vi "Test U8 Comm.vi"() -> ()   [LabVIEW 2021]
uses:
  ChannelCommon/typedef/FIFO Config.ctl
  ChannelCommon/ChannelCommon.lvlib
  CIFChannels/Typedef/Direction.ctl
  CIFChannels/CIFChannels.lvclass
  CIF_CIPC_Fifo_DAQ.lvclass
  ChannelCommon/typedef/TimeStamps.ctl
panel:
  out "status":string
  out "pass":bool
  out "error out":errorcluster
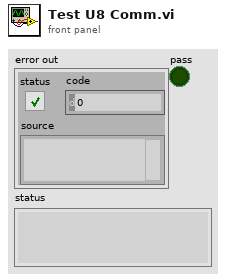
[diagram p1: front panel]
types:
  T1 = typedef "CIFChannels.lvclass/Direction.ctl" = enum16{"Publisher", "Subscriber"}
  T2 = typedef "ChannelCommon.lvlib/TimeStamps.ctl" = cluster{"ClockID":u8, "T0":i64, "T_Out":i64}
  T3 = typedef "ChannelCommon.lvlib/FIFO Config.ctl" = cluster{"Max Bytes/Msg":u64, "Max Msg/FIFO":u64, "Flags":u64}
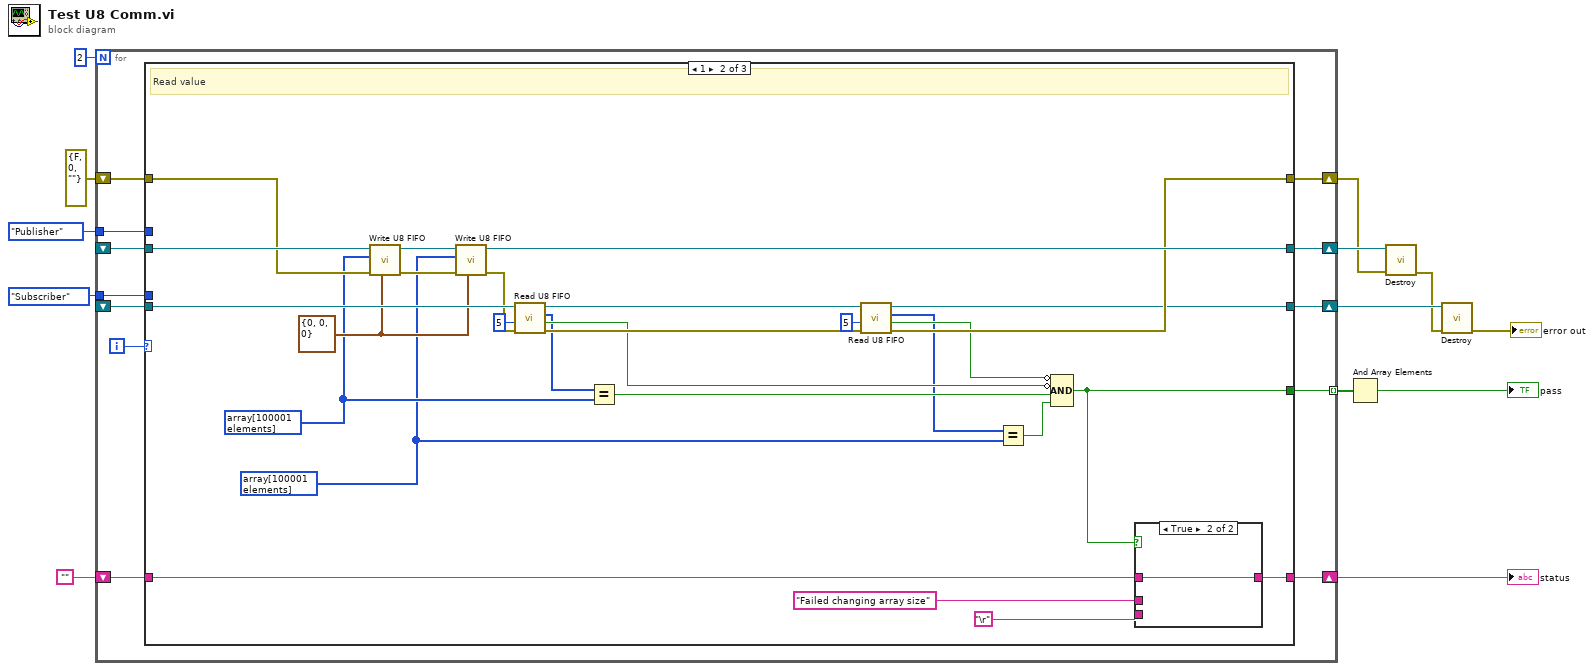
[diagram p0: block diagram]
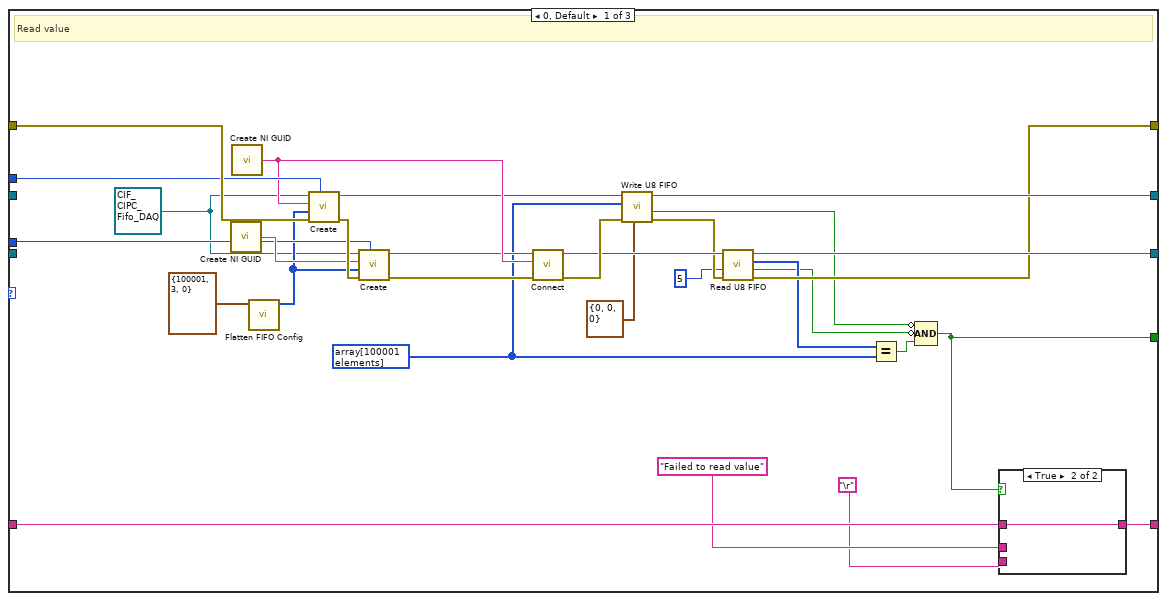
[diagram p2: hidden frame]
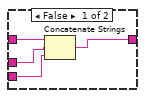
[diagram p3: hidden frame]
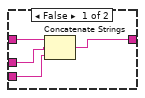
[diagram p4: hidden frame]
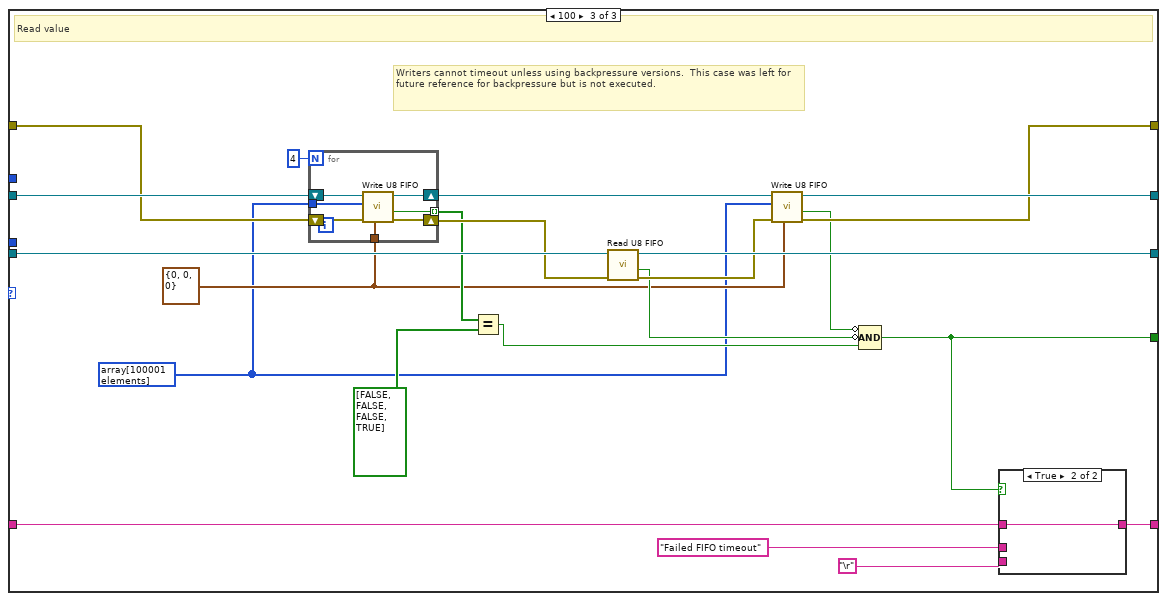
[diagram p5: hidden frame]
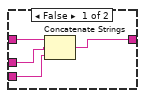
[diagram p6: hidden frame]
diagram:
  n1 = for {
    N: 2 -> [_]
    tunnel: [w25] -> w13 mode=indexing
    shift-right: [w23] -> w3
    shift-left: errorcluster {"status"=FALSE, "code"=0, "source"=""} ("error out") -> [w24]
    shift-right: [w20] -> w9
    shift-left: "" -> [w21]
    tunnel: Direction."Subscriber" ("Direction") -> [w19]
    tunnel: Direction."Publisher" ("Direction") -> [w18]
    shift-right: [w17] -> w5
    shift-left: _ -> [w15]
    shift-right: [w16] -> w4
    shift-left: _ -> [w14]
    i -> [w22]
    n2 = case shown="1" w22 {
      tunnel: [w50 w83 w95] -> w25
      tunnel: w24 -> [w48 w79 w109]
      tunnel: [w36 w72 w101] -> w23
      tunnel: w21 -> [w55 w87 w114]
      tunnel: [w54 w86 w113] -> w20
      tunnel: w19 -> [w46 _ _]
      tunnel: w18 -> [w45 _ _]
      tunnel: [w37 w69 w106] -> w17
      tunnel: [w39 w76 w104] -> w16
      tunnel: w14 -> [_ w80 w110]
      tunnel: w15 -> [_ w75 w107]
      frame 0, Default {
        w28 = refnum<class "CIF_CIPC_Fifo_DAQ.lvclass"> refnum ("CIF_CIPC_Fifo_U8.lvclass")
        w29 = u8[] array[100001 elements] ("U8 Data")
        # "Read value"
        n3 = call <vilib>:"Create NI GUID.vi"() -> ("NI GUID"=w47:string)
        n4 = call <vilib>:"Create NI GUID.vi"() -> ("NI GUID"=w43:string)
        n5 = call "Flatten FIFO Config.vi"("FIFO Config in"=T3 {"Max Bytes/Msg"=100001, "Max Msg/FIFO"=3, "Flags"=0}) -> ("Flattened FIFO Config"=w30:u8[])  [unwired: 10 in]
        n6 = call-dynamic "Create.vi"("Direction"=w45, "error in (no error)"=w48, "Custom Config Data"=w30, "Name"=w43, "CIFFIFO in"=w28) -> ("error out"=w49:errorcluster, "CIFFIFO out"=w26:refnum<class "CIF_CIPC_Fifo_DAQ.lvclass">)  [unwired: 5 in]
        n7 = call-dynamic "Create.vi"("Direction"=w46, "error in (no error)"=w49, "Custom Config Data"=w30, "Name"=w47, "CIFFIFO in"=w28) -> ("error out"=w42:errorcluster, "CIFFIFO out"=w41:refnum<class "CIF_CIPC_Fifo_DAQ.lvclass">)  [unwired: 5 in]
        n8 = call-dynamic "Connect.vi"("error in (no error)"=w42, "Connection Name"=w43, "CIFTag in"=w41) -> ("error out"=w40:errorcluster, "CIFTag out"=w38:refnum<class "CIF_CIPC_Fifo_DAQ.lvclass">)  [unwired: 7 in]
        n9 = call-dynamic "Write U8 FIFO.vi"("FIFO Timestamps"=T2 {"ClockID"=0, "T0"=0, "T_Out"=0}, "error in (no error)"=w40, "Data in"=w29, "CIFFIFO in"=w26) -> ("error out"=w35:errorcluster, "timed out?"=w34:bool, "CIFFIFO out"=w39:refnum<class "CIF_CIPC_Fifo_DAQ.lvclass">)  [unwired: 4 in, 1 out]
        n10 = call-dynamic "Read U8 FIFO.vi"("error in (no error)"=w35, "Timeout (ms)"=5, "CIFFIFO in"=w38) -> ("error out"=w36:errorcluster, "timed out?"=w32:bool, "Data out"=w33:u8[], "CIFFIFO out"=w37:refnum<class "CIF_CIPC_Fifo_DAQ.lvclass">)  [unwired: 4 in, 1 out]
        n11 = Equal?(x=w33, y=w29) -> (x = y?=w51:bool)
        n12 = Compound Arithmetic op=AND(invert w34, invert w32, w51) -> (w50:bool)
        n13 = case shown="True" w50 {
          tunnel: w55 -> [w59 w60]
          tunnel: [w56 w60] -> w54
          tunnel: "Failed to read value" -> [w58 _]
          tunnel: "\r" -> [w57 _]
          frame False {
            n14 = Concatenate Strings(w59, w58, w57) -> (w56:string)
          }
          frame True {
          }
        }
      }
      frame 1 {
        w61 = u8[] array[100001 elements] ("U8 Data")
        w62 = u8[] array[100001 elements] ("U8 Data")
        w63 = T2 {"ClockID"=0, "T0"=0, "T_Out"=0} ("FIFO Timestamps")
        # "Read value"
        n15 = call-dynamic "Write U8 FIFO.vi"("FIFO Timestamps"=w63, "error in (no error)"=w79, "Data in"=w62, "CIFFIFO in"=w80) -> ("error out"=w77:errorcluster, "CIFFIFO out"=w78:refnum<class "CIF_CIPC_Fifo_DAQ.lvclass">)  [unwired: 4 in, 2 out]
        n16 = call-dynamic "Write U8 FIFO.vi"("FIFO Timestamps"=w63, "error in (no error)"=w77, "Data in"=w61, "CIFFIFO in"=w78) -> ("error out"=w73:errorcluster, "CIFFIFO out"=w76:refnum<class "CIF_CIPC_Fifo_DAQ.lvclass">)  [unwired: 4 in, 2 out]
        n17 = call-dynamic "Read U8 FIFO.vi"("error in (no error)"=w73, "Timeout (ms)"=5, "CIFFIFO in"=w75) -> ("error out"=w71:errorcluster, "timed out?"=w67:bool, "Data out"=w64:u8[], "CIFFIFO out"=w68:refnum<class "CIF_CIPC_Fifo_DAQ.lvclass">)  [unwired: 4 in, 1 out]
        n18 = Equal?(x=w64, y=w62) -> (x = y?=w81:bool)
        n19 = call-dynamic "Read U8 FIFO.vi"("error in (no error)"=w71, "Timeout (ms)"=5, "CIFFIFO in"=w68) -> ("error out"=w72:errorcluster, "timed out?"=w66:bool, "Data out"=w65:u8[], "CIFFIFO out"=w69:refnum<class "CIF_CIPC_Fifo_DAQ.lvclass">)  [unwired: 4 in, 1 out]
        n20 = Equal?(x=w65, y=w61) -> (x = y?=w82:bool)
        n21 = Compound Arithmetic op=AND(invert w66, invert w67, w81, w82) -> (w83:bool)
        n22 = case shown="True" w83 {
          tunnel: w87 -> [w91 w92]
          tunnel: [w88 w92] -> w86
          tunnel: "Failed changing array size" -> [w90 _]
          tunnel: "\r" -> [w89 _]
          frame False {
            n23 = Concatenate Strings(w91, w90, w89) -> (w88:string)
          }
          frame True {
          }
        }
      }
      frame 100 {
        w93 = u8[] array[100001 elements] ("U8 Data")
        w94 = T2 {"ClockID"=0, "T0"=0, "T_Out"=0} ("FIFO Timestamps")
        # "Writers cannot timeout unless using backpressure versions.  This case was left for future reference for backpressure but is not executed."
        # "Read value"
        n24 = for {
          N: 4 -> [_]
          tunnel: w93 -> [w119]
          tunnel: w94 -> [w118]
          shift-right: [w117] -> w105
          shift-left: w110 -> [w121]
          tunnel: [w116] -> w100 mode=indexing
          shift-right: [w115] -> w103
          shift-left: w109 -> [w120]
          n25 = call-dynamic "Write U8 FIFO.vi"("FIFO Timestamps"=w118, "error in (no error)"=w120, "Data in"=w119, "CIFFIFO in"=w121) -> ("error out"=w115:errorcluster, "timed out?"=w116:bool, "CIFFIFO out"=w117:refnum<class "CIF_CIPC_Fifo_DAQ.lvclass">)  [unwired: 4 in, 1 out]
        }
        n26 = Equal?(x=w100, y=bool[] [FALSE, FALSE, FALSE, TRUE]) -> (x = y?=w96:bool)
        n27 = call-dynamic "Read U8 FIFO.vi"("error in (no error)"=w103, "CIFFIFO in"=w107) -> ("error out"=w102:errorcluster, "timed out?"=w98:bool, "CIFFIFO out"=w106:refnum<class "CIF_CIPC_Fifo_DAQ.lvclass">)  [unwired: 5 in, 2 out]
        n28 = call-dynamic "Write U8 FIFO.vi"("FIFO Timestamps"=w94, "error in (no error)"=w102, "Data in"=w93, "CIFFIFO in"=w105) -> ("error out"=w101:errorcluster, "timed out?"=w97:bool, "CIFFIFO out"=w104:refnum<class "CIF_CIPC_Fifo_DAQ.lvclass">)  [unwired: 4 in, 1 out]
        n29 = Compound Arithmetic op=AND(invert w97, invert w98, w96) -> (w95:bool)
        n30 = case shown="True" w95 {
          tunnel: w114 -> [w125 w126]
          tunnel: [w122 w126] -> w113
          tunnel: "Failed FIFO timeout" -> [w124 _]
          tunnel: "\r" -> [w123 _]
          frame False {
            n31 = Concatenate Strings(w125, w124, w123) -> (w122:string)
          }
          frame True {
          }
        }
      }
    }
  }
  "status" <- w9
  n32 = And Array Elements(Boolean array=w13) -> (logical AND=→"pass":bool)
  n33 = call-dynamic "Destroy.vi"("error in (no error)"=w3, "CIFTag in"=w4) -> ("error out"=w2:errorcluster)  [unwired: 8 in, 1 out]
  n34 = call-dynamic "Destroy.vi"("error in (no error)"=w2, "CIFTag in"=w5) -> ("error out"=→"error out":errorcluster)  [unwired: 8 in, 1 out]
